vi "Readable String.vi"(11 "SeqLoaded Condition in":refnum<class "SeqLoaded Condition.lvclass">) -> (2 "String":string)   [LabVIEW 2020, in "VolatusSeq.lvlib" / "SeqLoaded Condition.lvclass"]
uses:
  SeqLoaded Condition.lvclass
  SeqLoaded Condition.lvclass/SeqLoaded Condition.ctl
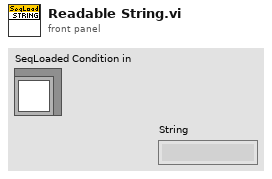
[diagram p1: front panel]
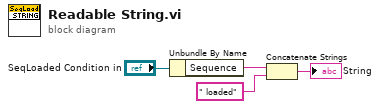
[diagram p0: block diagram]
diagram:
  n1 = Unbundle By Name("SeqLoaded Condition in") -> ("Sequence"=w3:string)
  n2 = Concatenate Strings(w3, " loaded" ("string")) -> (→"String":string)
